vi "Handshake_Test.vi"(8 "error in":errorcluster, 9 "Tester Tx":T2={"Fault"=FALSE, "StepNo"=0, "Ready"=TRUE, "HighVoltage"=FALSE, "TestRunning"=FALSE, "ResultsReady"=FALSE, "Results"=0, "ElapsedTime"=0, "Online"=TRUE, "TimeCompleted"=[], "Timeout"=FALSE, "Heartbeat"=FALSE}, 10 "Tester Rx In":T1={"Start"=FALSE, "NestStatus"=FALSE, "PalletID"=0, "BarcodeData"="P:10-000001R:04S:QMC2200001", "StepEcho"=0, "Cylinder_1"=FALSE, "Cylinder_2"=FALSE, "Cylinder_3"=FALSE, "Cylinder_4"=FALSE, "Cylinder_5"=FALSE, "ResultsAck"=FALSE, "Reset"=FALSE, "Stop"=FALSE, "FaultCode"=0}) -> (0 "error out":errorcluster, 2 "Tester Rx out":T1)   [LabVIEW 2019, in "Station Actor.lvlib" / "Station Actor.lvclass"]
uses:
  Station Actor.lvclass
  Custom Controls/Tester Rx Dataset.ctl
  Custom Controls/Tester Tx Dataset.ctl
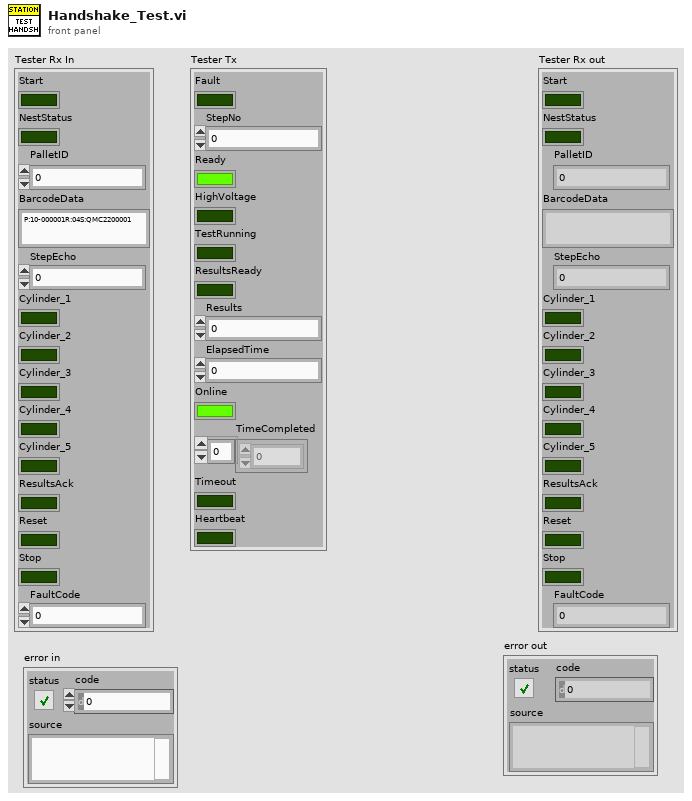
[diagram p1: front panel]
types:
  T1 = typedef "Station Actor.lvlib/Station Actor.lvclass/Tester Rx Dataset.ctl" = cluster{"Start":bool, "NestStatus":bool, "PalletID":u32, "BarcodeData":string, "StepEcho":u32, "Cylinder_1":bool, "Cylinder_2":bool, "Cylinder_3":bool, "Cylinder_4":bool, "Cylinder_5":bool, "ResultsAck":bool, "Reset":bool, "Stop":bool, "FaultCode":u32}
  T2 = typedef "Station Actor.lvlib/Station Actor.lvclass/Tester Tx Dataset.ctl" = cluster{"Fault":bool, "StepNo":u32, "Ready":bool, "HighVoltage":bool, "TestRunning":bool, "ResultsReady":bool, "Results":u32, "ElapsedTime":u32, "Online":bool, "TimeCompleted":i32[], "Timeout":bool, "Heartbeat":bool}
  T3 = cluster{"[0]":bool, "[1]":bool, "[2]":bool, "[3]":bool, "[4]":bool}
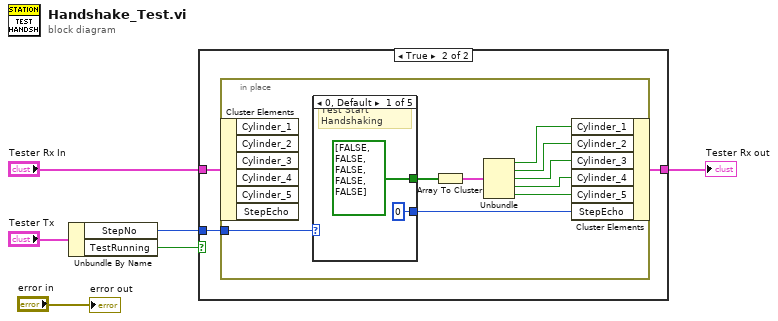
[diagram p0: block diagram]
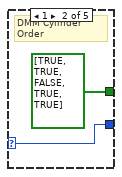
[diagram p3: hidden frame]
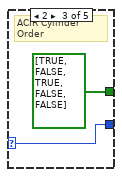
[diagram p4: hidden frame]
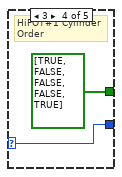
[diagram p5: hidden frame]
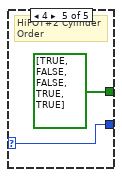
[diagram p6: hidden frame]
diagram:
  n1 = Unbundle By Name("Tester Tx") -> ("StepNo"=w1:u32, "TestRunning"=w5:bool)
  n2 = case shown="True" w5 {
    tunnel: "Tester Rx In" -> [w7 w10]
    tunnel: [w7 w9] -> w2
    tunnel: w1 -> [_ w8]
    frame False {
    }
    frame True {
      n3 = in-place {
        in-place-border: w8 -> [w19]
        n4 = in-place-cluster #1(w10) -> ()  [unwired: 6 out]
        n5 = case shown="0, Default" w19 {
          selector: w19 -> [_ w22 w24 w26 w28]
          tunnel: [bool[] [FALSE, FALSE, FALSE, FALSE, FALSE] bool[] [TRUE, TRUE, FALSE, TRUE, TRUE] bool[] [TRUE, FALSE, TRUE, FALSE, FALSE] bool[] [TRUE, FALSE, FALSE, FALSE, TRUE] bool[] [TRUE, FALSE, FALSE, TRUE, TRUE]] -> w18
          tunnel: [u32 0 ("StepNo") w22 w24 w26 w28] -> w11
          frame 0, Default {
            # "Test Start Handshaking"
          }
          frame 1 {
            # "DMM Cylinder Order"
          }
          frame 2 {
            # "ACIR Cylinder Order"
          }
          frame 3 {
            # "HiPOT#1 Cylinder Order"
          }
          frame 4 {
            # "HiPOT#2 Cylinder Order"
          }
        }
        n6 = Array To Cluster(array=w18) -> (cluster=w17:T3)
        n7 = Unbundle(w17) -> ("[0]"=w16:bool, "[1]"=w15:bool, "[2]"=w14:bool, "[3]"=w13:bool, "[4]"=w12:bool)
        n8 = in-place-cluster #1("Cylinder_1"=w16, "Cylinder_2"=w15, "Cylinder_3"=w14, "Cylinder_4"=w13, "Cylinder_5"=w12, "StepEcho"=w11) -> (w9:T1)
      }
    }
  }
  "Tester Rx out" <- w2
  "error out" <- "error in"
